vi "Read Sample Containers.vi"(11 "Storage Line in":refnum<class "Storage Line.lvclass">) -> (2 "Sample Containers":T1[](array[typedef])=[{"Sample In"="ni.var.psp://10.2.0.20/AMS Gas SHV/Storage Line/Tube 01/Sample In", "Sample Name"="ni.var.psp://10.2.0.20/AMS Gas SHV/Storage Line/Tube 01/Sample Name", "Ti Cathode"="ni.var.psp://10.2.0.20/AMS Gas SHV/Storage Line/Tube 01/Ti Cathode", "SampleQ"=refnum}, {"Sample In"="ni.var.psp://10.2.0.20/AMS Gas SHV/Storage Line/Tube 02/Sample In", "Sample Name"="ni.var.psp://10.2.0.20/AMS Gas SHV/Storage Line/Tube 02/Sample Name", "Ti Cathode"="ni.var.psp://10.2.0.20/AMS Gas SHV/Storage Line/Tube 02/Ti Cathode", "SampleQ"=refnum}, {"Sample In"="ni.var.psp://10.2.0.20/AMS Gas SHV/Storage Line/Tube 03/Sample In", "Sample Name"="ni.var.psp://10.2.0.20/AMS Gas SHV/Storage Line/Tube 03/Sample Name", "Ti Cathode"="ni.var.psp://10.2.0.20/AMS Gas SHV/Storage Line/Tube 03/Ti Cathode", "SampleQ"=refnum}, {"Sample In"="ni.var.psp://10.2.0.20/AMS Gas SHV/Storage Line/Tube 04/Sample In", "Sample Name"="ni.var.psp://10.2.0.20/AMS Gas SHV/Storage Line/Tube 04/Sample Name", "Ti Cathode"="ni.var.psp://10.2.0.20/AMS Gas SHV/Storage Line/Tube 04/Ti Cathode", "SampleQ"=refnum}, {"Sample In"="ni.var.psp://10.2.0.20/AMS Gas SHV/Storage Line/Tube 05/Sample In", "Sample Name"="ni.var.psp://10.2.0.20/AMS Gas SHV/Storage Line/Tube 05/Sample Name", "Ti Cathode"="ni.var.psp://10.2.0.20/AMS Gas SHV/Storage Line/Tube 05/Ti Cathode", "SampleQ"=refnum}, {"Sample In"="ni.var.psp://10.2.0.20/AMS Gas SHV/Storage Line/Tube 06/Sample In", "Sample Name"="ni.var.psp://10.2.0.20/AMS Gas SHV/Storage Line/Tube 06/Sample Name", "Ti Cathode"="ni.var.psp://10.2.0.20/AMS Gas SHV/Storage Line/Tube 06/Ti Cathode", "SampleQ"=refnum}, {"Sample In"="ni.var.psp://10.2.0.20/AMS Gas SHV/Storage Line/Tube 07/Sample In", "Sample Name"="ni.var.psp://10.2.0.20/AMS Gas SHV/Storage Line/Tube 07/Sample Name", "Ti Cathode"="ni.var.psp://10.2.0.20/AMS Gas SHV/Storage Line/Tube 07/Ti Cathode", "SampleQ"=refnum}, {"Sample In"="ni.var.psp://10.2.0.20/AMS Gas SHV/Storage Line/Tube 08/Sample In", "Sample Name"="ni.var.psp://10.2.0.20/AMS Gas SHV/Storage Line/Tube 08/Sample Name", "Ti Cathode"="ni.var.psp://10.2.0.20/AMS Gas SHV/Storage Line/Tube 08/Ti Cathode", "SampleQ"=refnum}, {"Sample In"="ni.var.psp://10.2.0.20/AMS Gas SHV/Storage Line/Tube 09/Sample In", "Sample Name"="ni.var.psp://10.2.0.20/AMS Gas SHV/Storage Line/Tube 09/Sample Name", "Ti Cathode"="ni.var.psp://10.2.0.20/AMS Gas SHV/Storage Line/Tube 09/Ti Cathode", "SampleQ"=refnum}, {"Sample In"="ni.var.psp://10.2.0.20/AMS Gas SHV/Storage Line/Tube 10/Sample In", "Sample Name"="ni.var.psp://10.2.0.20/AMS Gas SHV/Storage Line/Tube 10/Sample Name", "Ti Cathode"="ni.var.psp://10.2.0.20/AMS Gas SHV/Storage Line/Tube 10/Ti Cathode", "SampleQ"=refnum}, {"Sample In"="ni.var.psp://10.2.0.20/AMS Gas SHV/Storage Line/Tube 11/Sample In", "Sample Name"="ni.var.psp://10.2.0.20/AMS Gas SHV/Storage Line/Tube 11/Sample Name", "Ti Cathode"="ni.var.psp://10.2.0.20/AMS Gas SHV/Storage Line/Tube 11/Ti Cathode", "SampleQ"=refnum}, {"Sample In"="ni.var.psp://10.2.0.20/AMS Gas SHV/Storage Line/Tube 12/Sample In", "Sample Name"="ni.var.psp://10.2.0.20/AMS Gas SHV/Storage Line/Tube 12/Sample Name", "Ti Cathode"="ni.var.psp://10.2.0.20/AMS Gas SHV/Storage Line/Tube 12/Ti Cathode", "SampleQ"=refnum}], 3 "Storage Line out":refnum<class "Storage Line.lvclass">)   [LabVIEW 2015, in "cRIO-Carbondioxide.lvlib" / "CO2-Actor.lvlib" / "Storage Line.lvclass"]
uses:
  Storage Line.lvclass
  Controls/Sample Container.ctl
  subs/Sample/Sample.lvclass
  Storage Line.lvclass/Storage Line.ctl
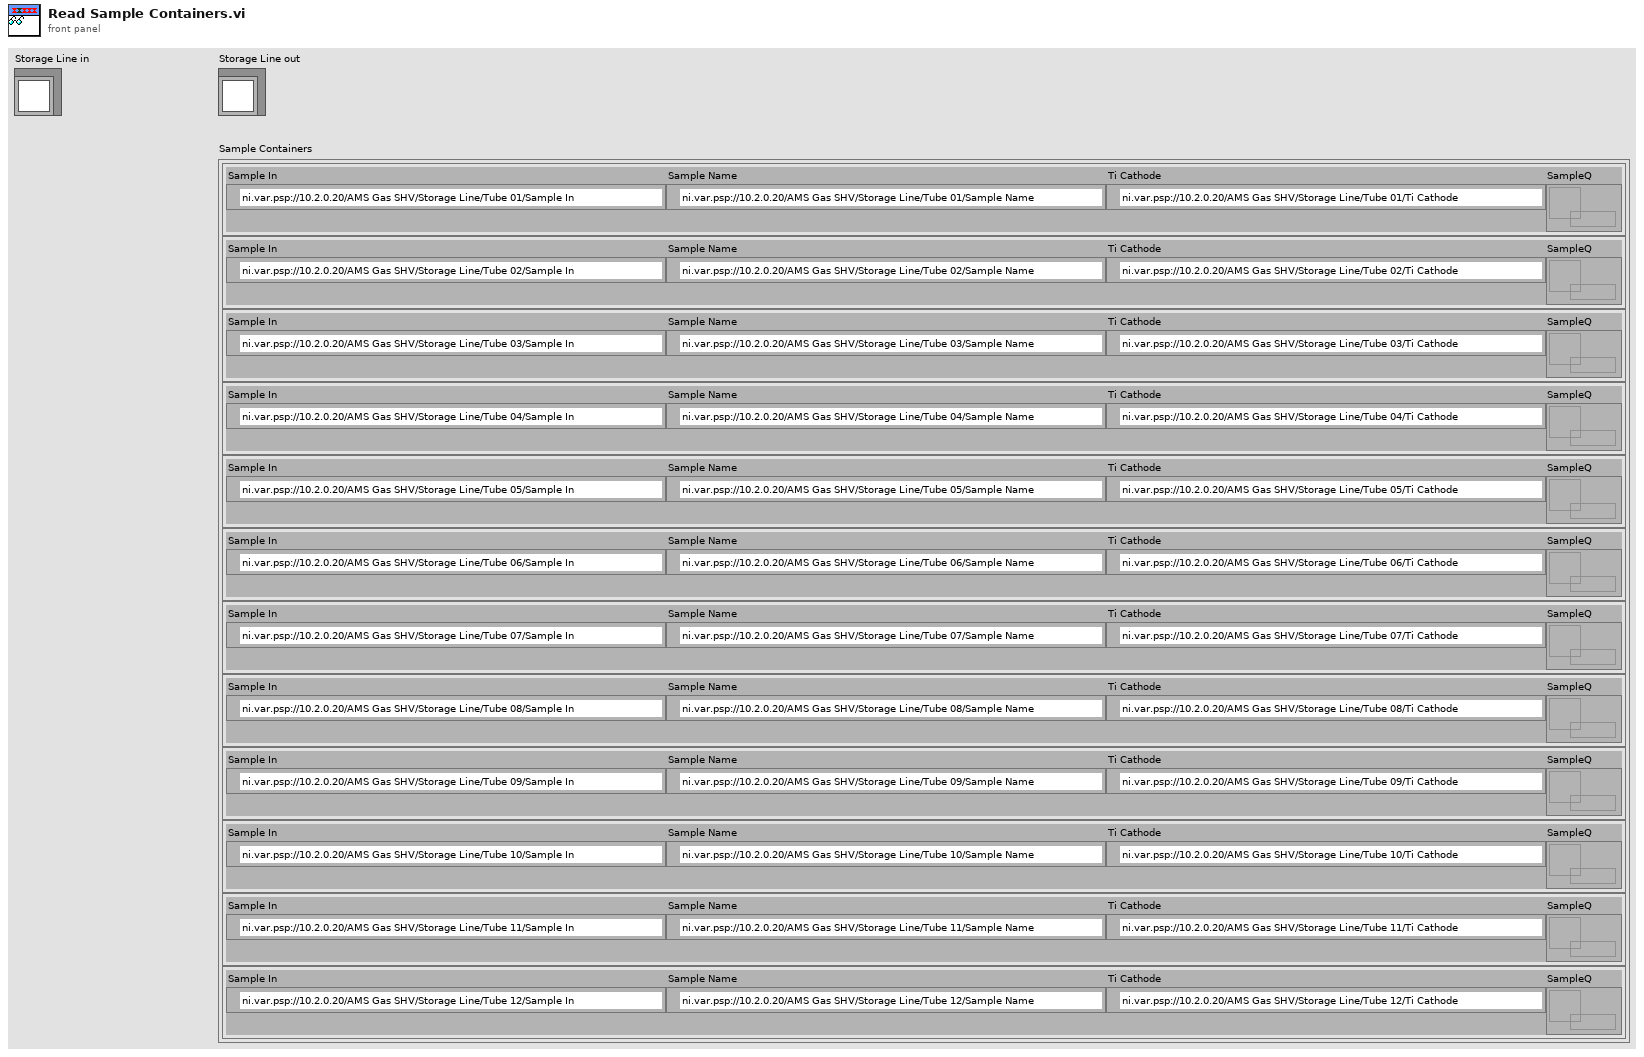
[diagram p1: front panel]
types:
  T1 = typedef "Sample Container.ctl" = cluster{"Sample In":refnum<k21>, "Sample Name":refnum<k21>, "Ti Cathode":refnum<k21>, "SampleQ":refnum<queue>}
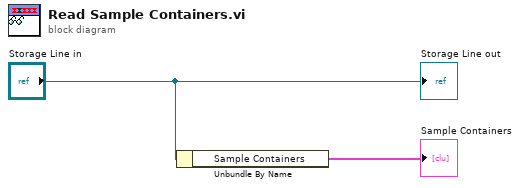
[diagram p0: block diagram]
diagram:
  n1 = Unbundle By Name("Storage Line in") -> ("Sample Containers"=→"Sample Containers":T1[])
  "Storage Line out" <- "Storage Line in"
